vi "Image.vi"(2 "XRef":refnum<vi>, 3 "State In":T1) -> (0 "Image":picture)   [LabVIEW 2018, in "ArrayDimension.xnode"]
uses:
  ArrayDimension.xnode
  State.ctl
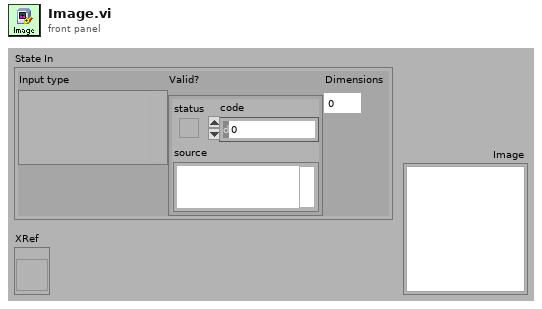
[diagram p1: front panel]
types:
  T1 = typedef "ArrayDimension.xnode/State.ctl" = cluster{"Input type":variant, "Valid?":errorcluster, "Dimensions":i32}
  T2 = typedef "imagedata.ctl" = cluster{"image type":i32, "image depth":i32, "image":u8[], "mask":u8[], "colors":u32[], "Rectangle":cluster{"left":i16, "top":i16, "right":i16, "bottom":i16}}
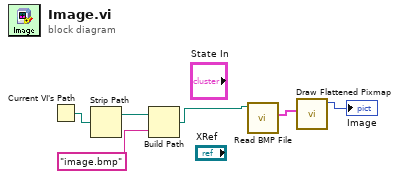
[diagram p0: block diagram]
diagram:
  n1 = Current VI's Path() -> (path=w6:path)
  n2 = Strip Path(path=w6) -> (stripped path=w5:path)  [unwired: 1 out]
  n3 = Build Path(base path=w5, name or relative path="image.bmp") -> (appended path=w3:path)
  n4 = call <vilib>:"Read BMP File.vi"("path to BMP file"=w3) -> ("image data"=w2:T2)  [unwired: 1 in, 9 out]
  n5 = call <vilib>:"Draw Flattened Pixmap.vi"("image data"=w2) -> ("new picture"=→"Image":picture)  [unwired: 1 in, 7 out]
